vi "Main.vi"() -> ()   [LabVIEW 2014]
doc: "This template is for the Queued Message Handler design pattern.\n\nThe Event Handling Loop generates messages based on user interface actions.\n\nThe Message Handling Loop processes messages generated by the Event Handling Loop, or by other messages. The messages are string values, so new messages can be added easily to the Message Cases case structure in the Message Handling Loop. Each message cluster can also provide an optional value for Message Data, which is a variant that can be converted to whatever message-specific data is required."
uses:
  Support/Type Definitions/UI Data.ctl
  support/Message Queue/Message Queue.lvlib
  Support/User Event - EHL Stop/User Event - EHL Stop.lvlib
  Support/Message Queue/Enqueue Message (Single).vi
  <vilib>/ErrorRing/Error Ring.xnode
  Model/Model.lvlib
  PLC/PLC.lvlib
  Support/Status Logger/Status Log.ctl
  <vilib>/Utility/error.llb/Error Cluster From Error Code.vi
  Support/Global names.vi
panel:
  out "Power status":bool
  in  "Abort":bool
  in  "Stop Line":bool
  in  "Start Line":bool
  out "Status":string
  in  "Tab Control":enum32{"Simulation"}(tab)
  in  "Power switch":bool
  in  "Positon":dbl(slide) scale=0.0..20.0
  in  "Dispose":bool
  in  "Pump":bool
  in  "Flow [l/s]":dbl=10.0
  in  "Exit":bool
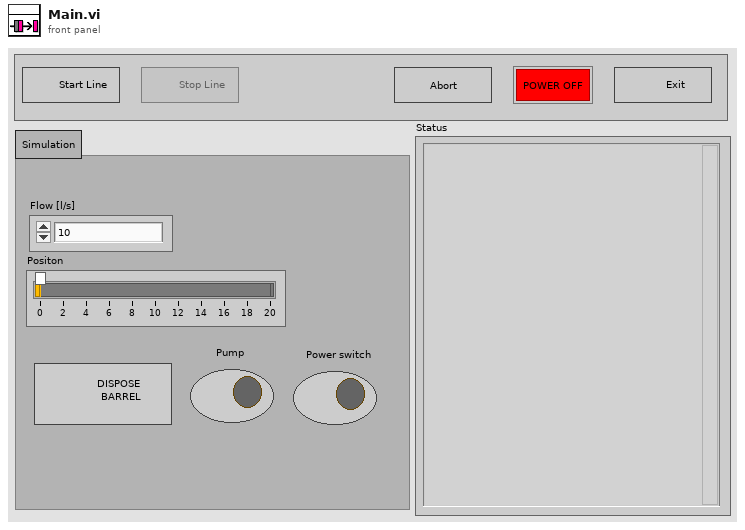
[diagram p1: front panel]
types:
  T1 = typedef "Status Log.ctl" = enum16{"Close file", "Open Status file", "Add Status", "Show Status File"}
  T2 = typedef "UI Data.ctl" = cluster{"Start Line Ref":refnum<vi>, "Stop Line Ref":refnum<vi>, "Data Display Ref":refnum<vi>, "Exit Button Ref":refnum<vi>, "Pump Ref":refnum<vi>, "Dispose Ref":refnum<vi>, "Flow Ref":refnum<vi>, "Position Ref":refnum<vi>, "Tab Ref":refnum<vi>, "Abort":refnum<vi>, "Power status":refnum<vi>, "Power switch":refnum<vi>}
  T3 = typedef "Notifiers.lvlib/Notifiers.ctl" = cluster{"PLC":refnum<notifier>, "Model":refnum<notifier>}
  T4 = typedef "Message Queue.lvlib/All Message Queues.ctl" = cluster{"UI":refnum<queue>, "Model":refnum<queue>, "PLC":refnum<queue>}
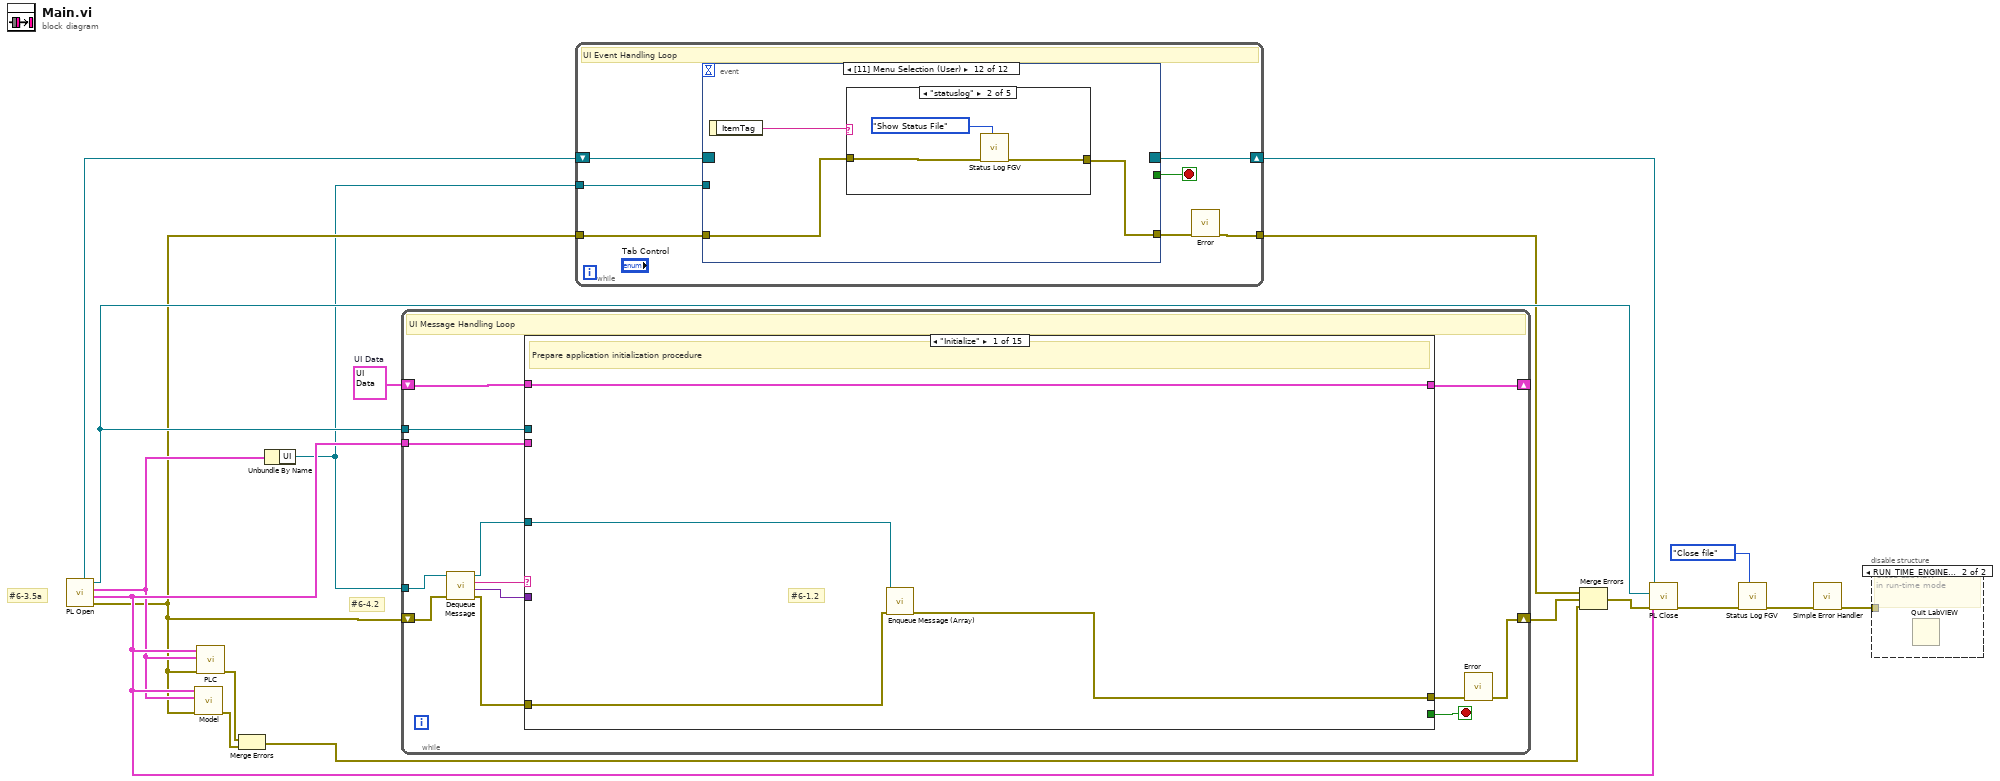
[diagram p0: block diagram]
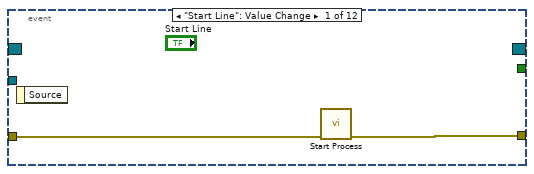
[diagram p2: hidden frame]
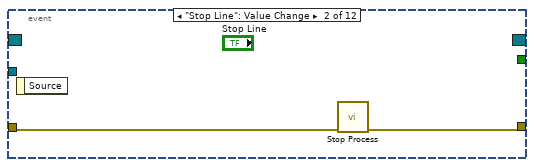
[diagram p3: hidden frame]
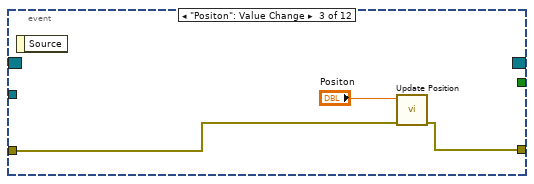
[diagram p4: hidden frame]
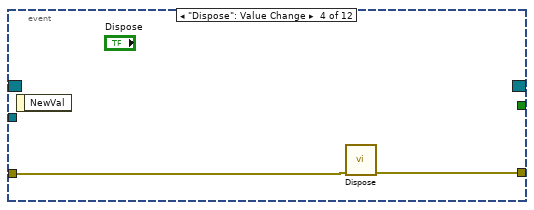
[diagram p5: hidden frame]
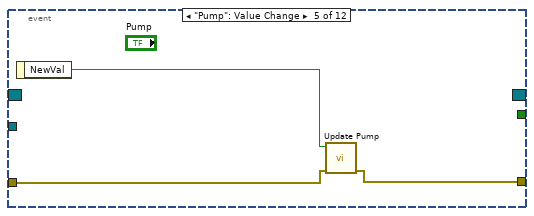
[diagram p6: hidden frame]
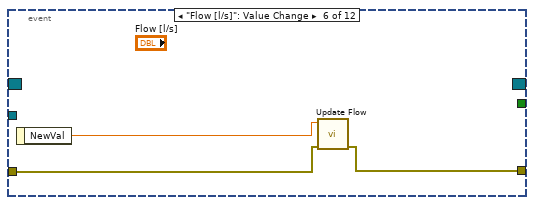
[diagram p7: hidden frame]
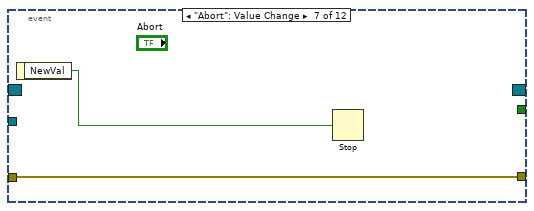
[diagram p8: hidden frame]
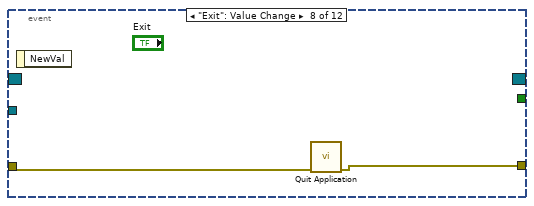
[diagram p9: hidden frame]
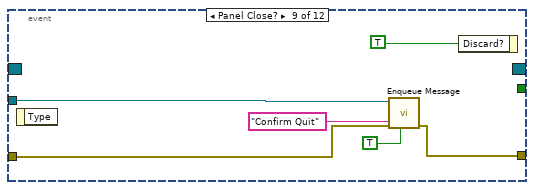
[diagram p10: hidden frame]
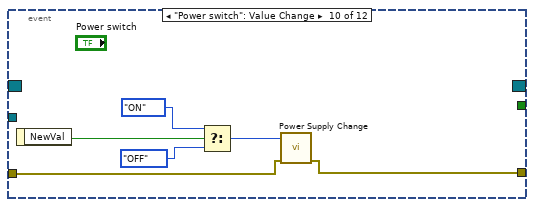
[diagram p11: hidden frame]
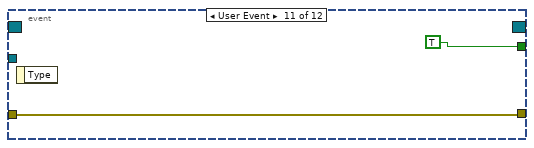
[diagram p12: hidden frame]
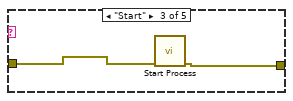
[diagram p14: hidden frame]
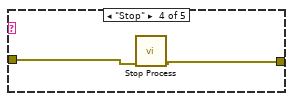
[diagram p15: hidden frame]
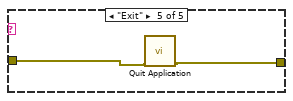
[diagram p16: hidden frame]
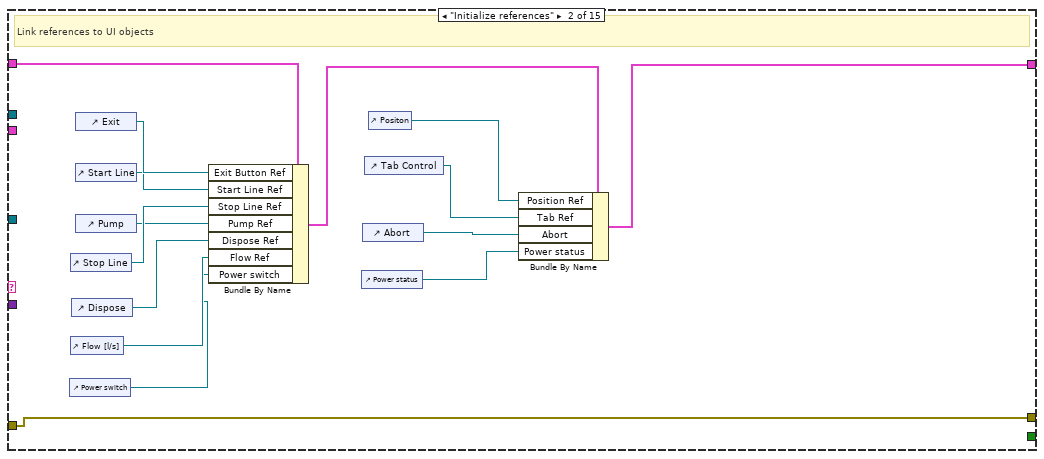
[diagram p18: hidden frame]
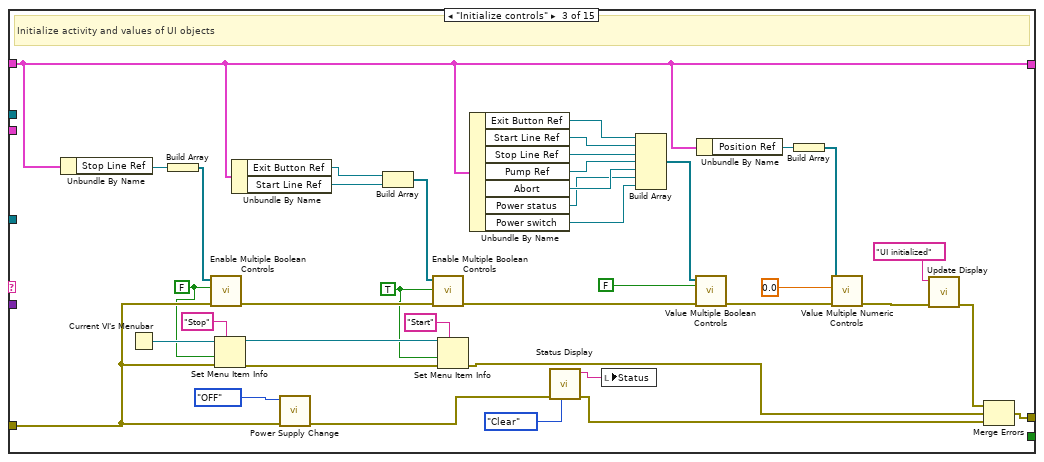
[diagram p19: hidden frame]
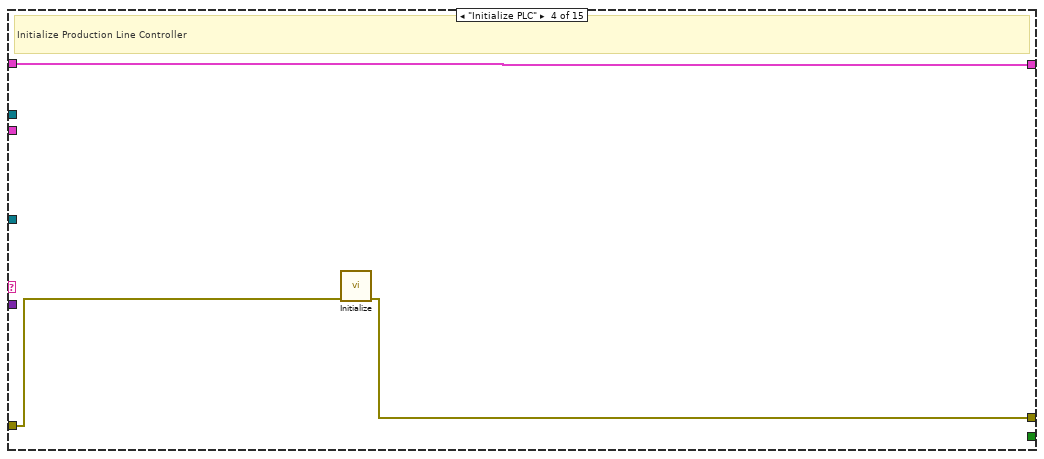
[diagram p20: hidden frame]
diagram:
  w17 = T2 {"Start Line Ref"=refnum, "Stop Line Ref"=refnum, "Data Display Ref"=refnum, "Exit Button Ref"=refnum, "Pump Ref"=refnum, "Dispose Ref"=refnum, "Flow Ref"=refnum, "Position Ref"=refnum, "Tab Ref"=refnum, "Abort"=refnum, "Power status"=refnum, "Power switch"=refnum}  # UI Data
  # "#6-3.5a"
  # "#6-4.2"
  n1 = call "PL Open.vi"() -> ("error out"=w2:errorcluster, "Notifiers"=w7:T3, "Queues"=w6:T4, "User Event"=w15:refnum<user-event>, "Event Registration Refnum"=w9:refnum<event-registration>)  [unwired: 7 in]
  n2 = call "Model.vi"("error in"=w2, "Queues"=w6, "Notifiers"=w7) -> ("error out"=w4:errorcluster)  [unwired: 8 in]
  n3 = call "PLC.vi"("error in"=w2, "Message Queues"=w6, "Notifiers"=w7) -> ("error out"=w5:errorcluster)  [unwired: 8 in]
  n4 = Merge Errors(w5, w4) -> (w3:errorcluster)
  n5 = Unbundle By Name(w6) -> ("UI"=w1:refnum<queue>)
  n6 = while {
    shift-right: [w30] -> _
    shift-left: w17 -> [w31]
    tunnel: w15 -> [w28]
    tunnel: w7 -> [w24]
    shift-right: [w20] -> w13
    shift-left: w2 -> [w27]
    tunnel: w1 -> [w22]
    stop <- w29 stop-if-true
    # "UI Message Handling Loop"
    n7 = call "Dequeue Message.vi"("error in (no error)"=w27, "Message Queue"=w22) -> ("error out"=w26:errorcluster, "Message Data"=w23:variant, "Message"=w19:string, "dup Message Queue"=w25:refnum<queue>)  [unwired: 6 in]
    n8 = case "Message Cases" shown="\"Initialize\"" w19 {
      selector: w19 -> [_ _ _ _ _ _ _ _ _ _ _ _ _ _ w244]
      tunnel: w25 -> [w33 _ _ _ _ _ _ _ _ _ w190 w196 w232 _ _]
      tunnel: w26 -> [w34 w39 w59 w90 w106 w124 w137 w152 w180 w182 w191 w198 w215 w239 _]
      tunnel: [w32 w39 w68 w91 w105 w126 w139 w153 w174 w181 w188 w195 w219 w233 w243] -> w21
      tunnel: w31 -> [w35 w50 w76 w92 w111 w136 w144 w156 w177 w186 w192 w202 w224 w238 w245]
      tunnel: [w35 w40 w76 w92 w111 w136 w144 w156 w177 w186 w192 w202 w224 w238 w245] -> w30
      tunnel: [_ _ _ _ _ _ _ _ _ _ _ _ TRUE _ _] -> w29
      tunnel: w23 -> [_ _ _ _ _ _ w147 w150 w179 w185 _ _ w226 _ _]
      tunnel: w28 -> [_ _ _ _ _ _ _ _ _ _ _ _ w229 _ _]
      tunnel: w24 -> [_ _ _ _ _ _ _ _ _ _ _ w201 _ _ _]
      frame "Initialize" {
        # "#6-1.2"
        # "Prepare application initialization procedure"
        n9 = call "Enqueue Message (Array).vi"("error in (no error)"=w34, "Message Queue"=w33) -> ("error out"=w32:errorcluster)  [unwired: 8 in, 1 out]
      }
      frame "Initialize references" {
        # "Link references to UI objects"
        n10 = control-ref of="Power switch"() -> (w38:refnum<vi>)
        n11 = control-ref of="Stop Line"() -> (w47:refnum<vi>)
        n12 = control-ref of="Flow [l/s]"() -> (w44:refnum<vi>)
        n13 = control-ref of="Dispose"() -> (w45:refnum<vi>)
        n14 = control-ref of="Exit"() -> (w49:refnum<vi>)
        n15 = control-ref of="Start Line"() -> (w48:refnum<vi>)
        n16 = control-ref of="Pump"() -> (w46:refnum<vi>)
        n17 = Bundle By Name(cluster=w50, "Exit Button Ref"=w49, "Start Line Ref"=w48, "Stop Line Ref"=w47, "Pump Ref"=w46, "Dispose Ref"=w45, "Flow Ref"=w44, "Power switch"=w38) -> (w43:T2)
        n18 = control-ref of="Power status"() -> (w36:refnum<vi>)
        n19 = control-ref of="Abort"() -> (w37:refnum<vi>)
        n20 = control-ref of="Tab Control"() -> (w41:refnum<vi>)
        n21 = control-ref of="Positon"() -> (w42:refnum<vi>)
        n22 = Bundle By Name(cluster=w43, "Position Ref"=w42, "Tab Ref"=w41, "Abort"=w37, "Power status"=w36) -> (w40:T2)
      }
      frame "Initialize controls" {
        w51 = TRUE ("Enabled")
        w52 = FALSE ("Enabled")
        # "Initialize activity and values of UI objects"
        n23 = Unbundle By Name(w76) -> ("Stop Line Ref"=w89:refnum<vi>)
        n24 = Current VI's Menubar() -> (w54:refnum<k9>)
        n25 = Build Array(w89) -> (w88:refnum<vi>[])
        n26 = call "Enable Multiple Boolean Controls.vi"("error in"=w59, "Enabled"=w52, "References"=w88) -> ("error out"=w85:errorcluster)  [unwired: 8 in]
        n27 = Set Menu Item Info(7:"Stop" ("item tag"), 8:w59, 9:w52, 11:w54) -> (0:w57:errorcluster, 3:w53:refnum<k9>)  [unwired: 3 in]
        n28 = Unbundle By Name(w76) -> ("Exit Button Ref"=w87:refnum<vi>, "Start Line Ref"=w86:refnum<vi>)
        n29 = call "Power Supply Change.vi"("error in"=w59, "Power status"=enum16{"OFF", "ON"}."OFF") -> ("error out"=w65:errorcluster)  [unwired: 9 in]
        n30 = Build Array(w87, w86) -> (w84:refnum<vi>[])
        n31 = call "Enable Multiple Boolean Controls.vi"("error in"=w85, "Enabled"=w51, "References"=w84) -> ("error out"=w79:errorcluster)  [unwired: 8 in]
        n32 = Set Menu Item Info(7:"Start" ("item tag"), 8:w57, 9:w51, 11:w53) -> (0:w55:errorcluster)  [unwired: 3 in, 1 out]
        n33 = Unbundle By Name(w76) -> ("Exit Button Ref"=w83:refnum<vi>, "Start Line Ref"=w82:refnum<vi>, "Stop Line Ref"=w81:refnum<vi>, "Pump Ref"=w80:refnum<vi>, "Abort"=w71:refnum<vi>, "Power status"=w70:refnum<vi>, "Power switch"=w61:refnum<vi>)
        n34 = call "Status Display.vi"("Action"=enum16{"Update", "Clear"}."Clear", "error in"=w65) -> ("error out"=w64:errorcluster, "Status"=w62:string)  [unwired: 8 in]
        n35 = local write "Status"(w62) -> ()
        n36 = Build Array(w83, w82, w81, w80, w71, w70, w61) -> (w77:refnum<vi>[])
        n37 = call "Value Multiple Boolean Controls.vi"("error in"=w79, "Value"=FALSE ("Enabled"), "References"=w77) -> ("error out"=w75:errorcluster)  [unwired: 8 in]
        n38 = Unbundle By Name(w76) -> ("Position Ref"=w74:refnum<vi>)
        n39 = Build Array(w74) -> (w73:refnum<vi>[])
        n40 = call "Value Multiple Numeric Controls.vi"("error in"=w75, "Value"=0.0, "References"=w73) -> ("error out"=w67:errorcluster)  [unwired: 8 in]
        n41 = call "Update Display.vi"("error in"=w67, "Message string"="UI initialized") -> ("error out"=w56:errorcluster)  [unwired: 9 in]
        n42 = Merge Errors(w56, w55, w64) -> (w68:errorcluster)
      }
      frame "Initialize PLC" {
        # "Initialize Production Line Controller"
        n43 = call "Initialize.vi"("error in"=w90) -> ("error out"=w91:errorcluster)  [unwired: 10 in]
      }
      frame "Start process" {
        w97 = TRUE ("Enabled")
        w101 = FALSE ("Enabled")
        # "Starts process: start PLC, open logger file, create reports files, enable/disable UI controls and update status display"
        n44 = Unbundle By Name(w111) -> ("Exit Button Ref"=w94:refnum<vi>, "Start Line Ref"=w107:refnum<vi>, "Stop Line Ref"=w110:refnum<vi>)
        n45 = Build Array(w94, w107) -> (w112:refnum<vi>[])
        n46 = Build Array(w110) -> (w109:refnum<vi>[])
        n47 = call "Start.vi"("error in"=w106) -> ("error out"=w108:errorcluster)  [unwired: 10 in]
        n48 = call "Enable Multiple Boolean Controls.vi"("error in"=w106, "Enabled"=w97, "References"=w109) -> ("error out"=w99:errorcluster)  [unwired: 8 in]
        n49 = call "Enable Multiple Boolean Controls.vi"("error in"=w106, "Enabled"=w101, "References"=w112) -> ("error out"=w103:errorcluster)  [unwired: 8 in]
        n50 = global read "Global names.vi" "Starting"() -> (w95:string)
        n51 = Current VI's Menubar() -> (w96:refnum<k9>)
        n52 = call "Update Display.vi"("error in"=w108, "Message string"=w95) -> ("error out"=w93:errorcluster)  [unwired: 9 in]
        n53 = Set Menu Item Info(7:"Start" ("item tag"), 8:w103, 9:w101, 11:w96) -> (0:w102:errorcluster)  [unwired: 3 in, 1 out]
        n54 = Set Menu Item Info(7:"Stop" ("item tag"), 8:w99, 9:w97, 11:w96) -> (0:w98:errorcluster)  [unwired: 3 in, 1 out]
        n55 = Merge Errors(w93, w102, w98) -> (w105:errorcluster)
      }
      frame "Stop process" {
        w115 = FALSE ("Enabled")
        w116 = TRUE ("Enabled")
        # "Stops process: stop PLC, close logger file, save and close report files, enable/disable UI controls and update status display"
        n56 = Unbundle By Name(w136) -> ("Exit Button Ref"=w113:refnum<vi>, "Start Line Ref"=w129:refnum<vi>, "Stop Line Ref"=w135:refnum<vi>)
        n57 = call "Stop.vi"("error in"=w124) -> ("error out"=w131:errorcluster)  [unwired: 10 in]
        n58 = Build Array(w135) -> (w125:refnum<vi>[])
        n59 = Build Array(w113, w129) -> (w133:refnum<vi>[])
        n60 = global read "Global names.vi" "Stopping"() -> (w114:string)
        n61 = Build Array (concatenate)(w133, w125) -> (w132:refnum<vi>[])
        n62 = call "Enable Multiple Boolean Controls.vi"("error in"=w124, "Enabled"=w116, "References"=w133) -> ("error out"=w121:errorcluster)  [unwired: 8 in]
        n63 = call "Enable Multiple Boolean Controls.vi"("error in"=w124, "Enabled"=w115, "References"=w125) -> ("error out"=w128:errorcluster)  [unwired: 8 in]
        n64 = call "Value Multiple Boolean Controls.vi"("error in"=w124, "Value"=FALSE, "References"=w132) -> ("error out"=w127:errorcluster)  [unwired: 8 in]
        n65 = call "Update Display.vi"("error in"=w131, "Message string"=w114) -> ("error out"=w130:errorcluster)  [unwired: 9 in]
        n66 = Current VI's Menubar() -> (w122:refnum<k9>)
        n67 = Set Menu Item Info(7:"Start" ("item tag"), 8:w121, 9:w116, 11:w122) -> (0:w119:errorcluster, 3:w117:refnum<k9>)  [unwired: 3 in]
        n68 = Set Menu Item Info(7:"Stop" ("item tag"), 8:w119, 9:w115, 11:w117) -> (0:w118:errorcluster)  [unwired: 3 in, 1 out]
        n69 = Merge Errors(w130, w118, w128, w127) -> (w126:errorcluster)
      }
      frame "Update display" {
        # "#6-3.5b"
        # "Updates status display, status log file and word report file"
        n70 = Variant To Data(error in=w137, type="", Variant=w147) -> (data=w138:string, error out=w141:errorcluster)
        n71 = call "Status Display.vi"("Action"=enum16{"Update", "Clear"}."Update", "error in"=w141, "Status line"=w138) -> ("error out"=w140:errorcluster, "Status"=→"Status":string)  [unwired: 7 in]
        n72 = property on="Status" class="Str"("Text.Scroll Position"=-1) -> ()  [unwired: 2 in, 2 out]
        n73 = Merge Errors(w137, w140) -> (w139:errorcluster)
      }
      frame "Update position" {
        # "Programmatically update position of the barrel slider"
        n74 = Variant To Data(error in=w152, type=0.0 ("Value"), Variant=w150) -> (data=w148:dbl, error out=w151:errorcluster)
        n75 = Unbundle By Name(w156) -> ("Position Ref"=w155:refnum<vi>)
        n76 = Build Array(w155) -> (w154:refnum<vi>[])
        n77 = call "Value Multiple Numeric Controls.vi"("error in"=w151, "Value"=w148, "References"=w154) -> ("error out"=w153:errorcluster)  [unwired: 8 in]
      }
      frame "Power status change" {
        # "Update main switch LED and Start/Stop buttons according to power status change (DAQ DI)"
        n78 = Variant To Data(error in=w180, type=TRUE, Variant=w179) -> (data=w157:bool, error out=w161:errorcluster)
        "Power status" <- w157
        n79 = Unbundle By Name(w177) -> ("Start Line Ref"=w176:refnum<vi>, "Stop Line Ref"=w175:refnum<vi>)
        n80 = Build Array(w176) -> (w173:refnum<vi>[])
        n81 = Build Array(w175) -> (w170:refnum<vi>[])
        n82 = Build Array (concatenate)(w173, w170) -> (w172:refnum<vi>[])
        n83 = Current VI's Menubar() -> (w164:refnum<k9>)
        n84 = call "Enable Multiple Boolean Controls.vi"("error in"=w161, "Enabled"=w157, "References"=w173) -> ("error out"=w168:errorcluster)  [unwired: 8 in]
        n85 = Set Menu Item Info(7:"Start" ("item tag"), 8:w161, 9:w157, 11:w164) -> (0:w162:errorcluster, 3:w158:refnum<k9>)  [unwired: 3 in]
        n86 = call "Value Multiple Boolean Controls.vi"("error in"=w161, "Value"=FALSE, "References"=w172) -> ("error out"=w167:errorcluster)  [unwired: 8 in]
        n87 = call "Enable Multiple Boolean Controls.vi"("error in"=w161, "Enabled"=FALSE, "References"=w170) -> ("error out"=w166:errorcluster)  [unwired: 8 in]
        n88 = Set Menu Item Info(7:"Stop" ("item tag"), 8:w162, 9:FALSE ("enabled"), 11:w158) -> (0:w159:errorcluster)  [unwired: 3 in, 1 out]
        n89 = Merge Errors(w168, w167, w166, w159) -> (w174:errorcluster)
      }
      frame "Error" {
        # "Display error dialog box and quit application"
        n90 = Variant To Data(error in=w182, type=errorcluster {"status"=FALSE, "code"=0, "source"=""} ("error constant"), Variant=w185) -> (data=w183:errorcluster, error out=w181:errorcluster)
        n91 = call <vilib>:"Simple Error Handler.vi"("error in (no error)"=w183) -> ()  [unwired: 4 in, 5 out]
      }
      frame "Exit" {
        # "Start exit procedure: stop PLC, then send Exit message to PLC and go to PLC confirmation loop"
        n92 = Flush Queue(queue=w190, error in (no error)=w191) -> (error out=w187:errorcluster)  [unwired: 2 out]
        n93 = call "Exit PLC.vi"("error in"=w187) -> ("error out"=w189:errorcluster)  [unwired: 10 in]
        n94 = call "Wait on PLC Exit.vi"("error in"=w189) -> ("error out"=w188:errorcluster)  [unwired: 10 in]
      }
      frame "Wait on PLC exit" {
        # "Wait until PLC shutdown"
        n95 = Unbundle By Name(w201) -> ("PLC"=w200:refnum<notifier>)
        n96 = Wait on Notification(notifier=w200, timeout in ms (-1)=10, error in (no error)=w198) -> (notification=w194:string, timed out?=w197:bool, error out=w193:errorcluster)  [unwired: 1 in, 1 out]
        n97 = case shown="True" w197 {
          tunnel: [w203 w212] -> w195
          tunnel: w193 -> [w204 w209]
          tunnel: w196 -> [_ w210]
          tunnel: w194 -> [_ w205]
          frame True {
            # "Shutdown notification from PLC not received"
            n98 = call "Wait on PLC Exit.vi"("error in"=w204) -> ("error out"=w203:errorcluster)  [unwired: 10 in]
          }
          frame False {
            # "Shutdown notification from PLC received (handshake)"
            n99 = call "Update Display.vi"("error in"=w209, "Message string"=w205) -> ("error out"=w208:errorcluster)  [unwired: 9 in]
            n100 = call "Update Display.vi"("error in"=w208, "Message string"="Application quits" ("Message")) -> ("error out"=w207:errorcluster)  [unwired: 9 in]
            n101 = call-poly "Enqueue Message.vi"("error in (no error)"=w207, "Message"="End program", "Message Queue"=w210) -> ("error out"=w212:errorcluster)  [unwired: 7 in, 1 out]
          }
        }
      }
      frame "End program" {
        # "Shutdown MHL and send exit user event to EHL; reset UI controls"
        n102 = call "Fire User Event - EHL Stop.vi"("error in (no error)"=w215, "User Event - Stop"=w229) -> ("error out"=w214:errorcluster)  [unwired: 9 in]
        n103 = Variant To Data(error in=w215, type=errorcluster {"status"=FALSE, "code"=0, "source"=""} ("error constant"), Variant=w226) -> (data=w227:errorcluster)  [unwired: 1 out]
        n104 = Release Queue(queue=w232, force destroy? (F)=TRUE, error in (no error)=w215) -> (error out=w230:errorcluster)  [unwired: 2 out]
        n105 = call <vilib>:"Simple Error Handler.vi"("error in (no error)"=w227) -> ("error out"=w213:errorcluster)  [unwired: 4 in, 4 out]
        n106 = Merge Errors(w214, w213, w230) -> (w220:errorcluster)
        n107 = Unbundle By Name(w224) -> ("Exit Button Ref"=w223:refnum<vi>, "Abort"=w218:refnum<vi>, "Start Line Ref"=w217:refnum<vi>, "Stop Line Ref"=w216:refnum<vi>)
        n108 = Build Array(w223, w218, w217, w216) -> (w222:refnum<vi>[])
        n109 = call "Value Multiple Boolean Controls.vi"("error in"=w220, "Value"=FALSE, "References"=w222) -> ("error out"=w219:errorcluster)  [unwired: 8 in]
      }
      frame "Confirm Quit" {
        # "Confirm Quit - Message that can confirm whether or not the user wants to exit the application."
        n110 = Two Button Dialog(message="Are you sure?", 1:"Continue" ("F button name (\"Cancel\")"), 2:"Quit" ("T button name (\"OK\")")) -> (T button?=w234:bool)
        n111 = case shown="True" w234 {
          tunnel: w239 -> [w240 w242]
          tunnel: [w240 w241] -> w233
          frame False {
          }
          frame True {
            n112 = call "Quit Application.vi"("error in"=w242) -> ("error out"=w241:errorcluster)  [unwired: 10 in]
          }
        }
      }
      frame Default {
        # "Incorrect message: show error and clear error"
        n113 = xnode "Error Ring"("parameter 0"=w244) -> ("error out"=w243:errorcluster)
      }
    }
    n114 = call "Error.vi"("error in"=w21) -> ("error out"=w20:errorcluster)  [unwired: 10 in]
  }
  n115 = while {
    tunnel: w1 -> [w255]
    shift-right: [w258] -> w18
    shift-left: w9 -> [w259]
    tunnel: [w253] -> w8
    tunnel: w2 -> [w256]
    stop <- w257 stop-if-true
    # "UI Event Handling Loop"
    n116 = event shown="[11] Menu Selection (User)" {
      selector: w259 -> [_ _ _ _ _ _ _ _ _ _ _ _]
      dyn-events: [_ _ _ _ _ _ _ _ _ _ _ _] -> w258
      timeout: _ -> [_ _ _ _ _ _ _ _ _ _ _ _]
      tunnel: [_ _ _ _ _ _ _ _ _ _ TRUE ("Discard?") _] -> w257
      tunnel: w255 -> [_ _ _ _ _ _ _ _ w284 _ _ _]
      tunnel: [w260 w262 w265 w267 w270 w273 w276 w277 w283 w285 w291 w294] -> w254
      tunnel: w256 -> [w261 w263 w264 w268 w271 w274 w276 w278 w279 w286 w291 w293]
      event "Start Line": Value Change {
        n117 = event-data() -> ()  [unwired: 1 in, 1 out]
        n118 = call "Start Process.vi"("error in"=w261) -> ("error out"=w260:errorcluster)  [unwired: 10 in]
      }
      event "Stop Line": Value Change {
        n119 = event-data() -> ()  [unwired: 1 in, 1 out]
        n120 = call "Stop Process.vi"("error in"=w263) -> ("error out"=w262:errorcluster)  [unwired: 10 in]
      }
      event "Positon": Value Change {
        n121 = event-data() -> ()  [unwired: 1 in, 1 out]
        n122 = call "Update Position.vi"("error in (no error)"=w264, "Position"="Positon") -> ("error out"=w265:errorcluster)  [unwired: 9 in]
      }
      event "Dispose": Value Change {
        n123 = event-data() -> ()  [unwired: 1 in, 1 out]
        n124 = call "Dispose.vi"("error in (no error)"=w268) -> ("error out"=w267:errorcluster)  [unwired: 10 in]
      }
      event "Pump": Value Change {
        n125 = event-data() -> ("NewVal"=w269:bool)  [unwired: 1 in]
        n126 = call "Update Pump.vi"("error in (no error)"=w271, "Pump State"=w269) -> ("error out"=w270:errorcluster)  [unwired: 9 in]
      }
      event "Flow [l/s]": Value Change {
        n127 = event-data() -> ("NewVal"=w272:dbl)  [unwired: 1 in]
        n128 = call "Update Flow.vi"("error in (no error)"=w274, "Flow"=w272) -> ("error out"=w273:errorcluster)  [unwired: 9 in]
      }
      event "Abort": Value Change {
        n129 = event-data() -> ("NewVal"=w275:bool)  [unwired: 1 in]
        n130 = Stop(stop? (T)=w275) -> ()
      }
      event "Exit": Value Change {
        n131 = event-data() -> ()  [unwired: 1 in, 1 out]
        n132 = call "Quit Application.vi"("error in"=w278) -> ("error out"=w277:errorcluster)  [unwired: 10 in]
      }
      event Panel Close? {
        n133 = event-data() -> ()  [unwired: 1 in, 1 out]
        n134 = call-poly "Enqueue Message.vi"("Priority Message? (F)"=TRUE, "error in (no error)"=w279, "Message"="Confirm Quit", "Message Queue"=w284) -> ("error out"=w283:errorcluster)  [unwired: 6 in, 1 out]
        n135 = event-data("Discard?"=TRUE) -> ()  [unwired: 1 in, 1 out]
      }
      event "Power switch": Value Change {
        n136 = event-data() -> ("NewVal"=w290:bool)  [unwired: 1 in]
        n137 = Select(t=enum16{"OFF", "ON"}."ON" ("Power status"), s=w290, f=enum16{"OFF", "ON"}."OFF" ("Power status")) -> (s? t:f=w287:enum16{"OFF", "ON"})
        n138 = call "Power Supply Change.vi"("error in"=w286, "Power status"=w287) -> ("error out"=w285:errorcluster)  [unwired: 9 in]
      }
      event User Event {
        n139 = event-data() -> ()  [unwired: 1 in, 1 out]
      }
      event Menu Selection (User) {
        n140 = event-data() -> ("ItemTag"=w295:string)  [unwired: 1 in]
        n141 = case shown="\"statuslog\"" w295 {
          tunnel: [w296 w297 w301 w302 w304] -> w294
          tunnel: w293 -> [w296 w298 w300 w303 w305]
          frame Default {
          }
          frame "statuslog" {
            n142 = call "Status Log FGV.vi"("Action"=Status_Log."Show Status File", "error in"=w298) -> ("error out"=w297:errorcluster)  [unwired: 9 in]
          }
          frame "Start" {
            n143 = call "Start Process.vi"("error in"=w300) -> ("error out"=w301:errorcluster)  [unwired: 10 in]
          }
          frame "Stop" {
            n144 = call "Stop Process.vi"("error in"=w303) -> ("error out"=w302:errorcluster)  [unwired: 10 in]
          }
          frame "Exit" {
            n145 = call "Quit Application.vi"("error in"=w305) -> ("error out"=w304:errorcluster)  [unwired: 10 in]
          }
        }
      }
    }
    n146 = call "Error.vi"("error in"=w254) -> ("error out"=w253:errorcluster)  [unwired: 10 in]
  }
  n147 = Merge Errors(w8, w13, w3) -> (w12:errorcluster)
  n148 = call "PL Close.vi"("error in"=w12, "Notifiers"=w7, "User Event"=w15, "Event Registration Refnum in"=w18) -> ("error out"=w16:errorcluster)  [unwired: 7 in]
  n149 = call "Status Log FGV.vi"("Action"=Status_Log."Close file", "error in"=w16) -> ("error out"=w10:errorcluster)  [unwired: 9 in]
  n150 = call <vilib>:"Simple Error Handler.vi"("error in (no error)"=w10) -> ("error out"=w11:errorcluster)  [unwired: 4 in, 4 out]
  n151 = disable-structure shown="RUN_TIME_ENGINE==True" {
    disable-tunnel: w11 -> [_ _]
    frame condition #0 (active) {
    }
    frame condition #1 {
      # "Close LabVIEW\nin run-time mode"
      n152 = Quit LabVIEW() -> ()  [unwired: 1 in]
    }
  }
